vi "BRig_dataExp_TPB_max_R.vi"() -> (2 "output_TPB_max_R":i32)   [LabVIEW 2014]
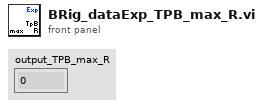
[diagram p1: front panel]
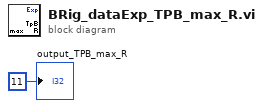
[diagram p0: block diagram]
diagram:
  "output_TPB_max_R" <- 11 ("output_iBlock")
